vi "draw.vi"(0 "new position":cluster{"x":i16, "y":i16}, 1 "L 1":dbl(slide)=80.0 scale=0.0..200.0, 2 "L 2":dbl(slide)=115.0 scale=0.0..200.0, 3 "Angle1":dbl(knob)=-45.83837436417874 scale=-90.0..90.0, 4 "Angle 2":dbl(knob)=-72.06882847083946 scale=-90.0..90.0, 5 "input pic in loop":picture, 7 "bias":dbl) -> (14 "end effector":cluster{dbl, dbl}={159.01647214211073, 1.9100783062530127} {"?" format="%.1f"; "?" format="%#.1f"}, 15 "mag":dbl, 16 "angle":dbl, 17 "2D Picture":picture, 18 "shift pic":picture)   [LabVIEW 2024]
panel:
  # "A 2"
  # "L1"
  # "L2"
  # "A 1"
  # "mm"
  # "mm"
  # "mm"
  # "mm"
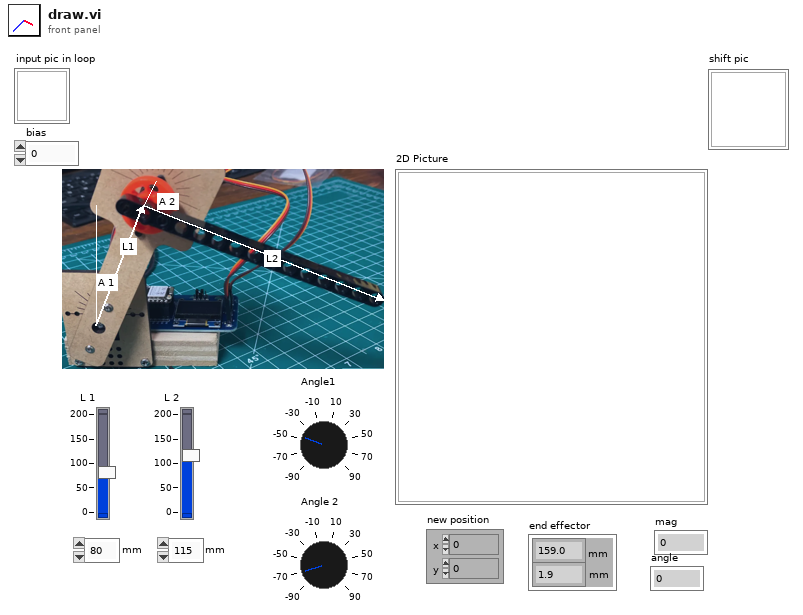
[diagram p1: front panel]
types:
  T1 = cluster{"Width":u16, "Style":enum32{"Solid", "Dash", "Dot", "DashDot", "DashDotDot"}}
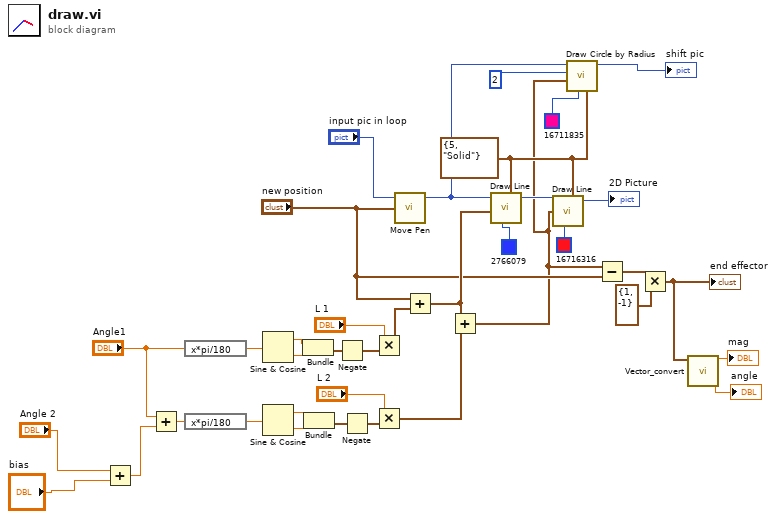
[diagram p0: block diagram]
diagram:
  w10 = T1 {"Width"=5, "Style"=enum."Solid"} ("pen")
  n1 = Add(x="Angle 2", y="bias") -> (x+y=w3:dbl)
  n2 = Add(x="Angle1", y=w3) -> (x+y=w27:dbl)
  n3 = expression code="x*pi/180"("Angle1") -> (w37:dbl)
  n4 = expression code="x*pi/180"(w27) -> (w33:dbl)
  n5 = Sine & Cosine(0:w37) -> (1:w20:dbl, 2:w19:dbl)
  n6 = Sine & Cosine(0:w33) -> (1:w17:dbl, 2:w16:dbl)
  n7 = Bundle(w20, w19) -> (w36:cluster{dbl, dbl})  [unwired: 1 in]
  n8 = Bundle(w17, w16) -> (w34:cluster{dbl, dbl})  [unwired: 1 in]
  n9 = Negate(x=w36) -> (-x=w18:cluster{dbl, dbl})
  n10 = Negate(x=w34) -> (-x=w15:cluster{dbl, dbl})
  n11 = Multiply(x="L 1", y=w18) -> (x*y=w35:cluster{dbl, dbl})
  n12 = Multiply(x="L 2", y=w15) -> (x*y=w31:cluster{dbl, dbl})
  n13 = call <vilib>:"Move Pen.vi"("new position"="new position", "picture"="input pic in loop") -> ("new picture"=w8:picture)  [unwired: 3 in]
  n14 = Add(x="new position", y=w35) -> (x+y=w30:cluster{dbl, dbl})
  n15 = Add(x=w31, y=w30) -> (x+y=w9:cluster{dbl, dbl})
  n16 = call <vilib>:"Draw Line.vi"("picture"=w8, "end point"=w30, "color(black)"=u32 2766079, "pen"=w10) -> ("new picture"=w32:picture)  [unwired: 5 in]
  n17 = call <vilib>:"Draw Line.vi"("picture"=w32, "end point"=w9, "color(black)"=u32 16716316, "pen"=w10) -> ("new picture"=→"2D Picture":picture)  [unwired: 5 in]
  n18 = call <vilib>:"Draw Circle by Radius.vi"("pen"=w10, "color(black)"=u32 16711835, "pixel center"=w9, "radius"=u16 2 ("Width"), "picture"=w8) -> ("new picture"=→"shift pic":picture)  [unwired: 6 in]
  n19 = Subtract(x=w9, y="new position") -> (x-y=w23:cluster{dbl, dbl})
  n20 = Multiply(x=w23, y=cluster{"x":i16, "y":i16} {"x"=1, "y"=-1} ("new position")) -> (x*y=w14:cluster{dbl, dbl})
  "end effector" <- w14
  n21 = call "Vector_convert.vi"("x,y"=w14) -> ("angle"=→"angle":dbl, "mag"=→"mag":dbl)  [unwired: 9 in]
